vi "OE2012&OE2022_Configure Demodulator Filter.vi"(7 "OE2012&OE2022_\nConfigure Demod Filter":T1={"Time Constant(s) "=0.1, "Low Pass Filter Slope "=1, "Enable Sync Filter "=0, "Demodulator Source"=0, "Demodulator"=1} {"Demodulator" items=["Demod1"=1, "Demod2"=2, "Demod3"=3, "Demod4"=4, "Demod5"=5, "Demod6"=6, "Demod7"=7, "Demod8"=8]; "Demodulator Source" items=["Signal In 1", "Signal In 2", "Aux In 1", "Aux In 2", "Aux In 3", "Aux In 4", "X-Demod1", "Y-Demod1", "R-Demod1", "Theta-Demod1", "X-Demod5", "Y-Demod5", "R-Demod5", "Theta-Demod5"]; "Enable Sync Filter" items=["OFF", "ON"]; "Low Pass Filter Slope" items=["6 dB/oct", "12 dB/oct", "18 db/oct", "24 dB/oct", "30 dB/oct", "36 dB/oct", "42 dB/oct", "48 dB/oct"]; "Time Constant(s)" min=1e-06 max=3000.0}, 8 "Error in (no error)":errorcluster caption="error out（no error）", 9 "Remote Mode":u16(ring)=1 items=["RS232"=1, "Ethernet"=3], 10 "Connection ID in":refnum<k5>, 11 "VISA resource name":refnum<visa-resource-name>) -> (0 "Error out":errorcluster caption="error out", 1 "Output String":string, 2 "Connection ID out":refnum<k5>, 3 "VISA resource  out":refnum<visa-resource-name>)   [LabVIEW 2011]
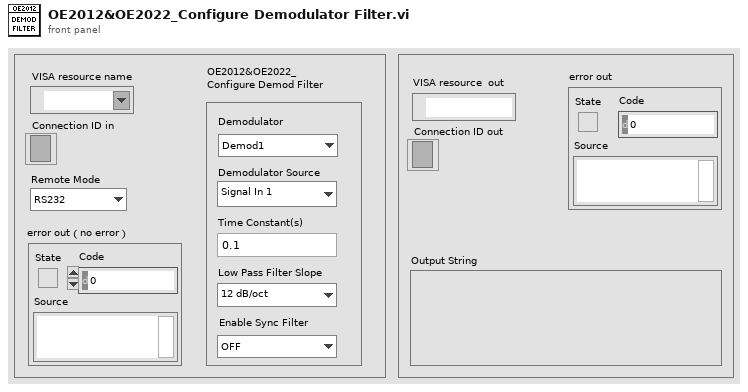
[diagram p1: front panel]
types:
  T1 = cluster{"Time Constant(s) ":dbl, "Low Pass Filter Slope ":u8, "Enable Sync Filter ":u16, "Demodulator Source":u16, "Demodulator":u16}
  T2 = enum16{"ISRC", "IGND", "ICPL", "ILIN", "PHAS", "FMOD", "RSLP", "FREQ", "SWPT", "SLLM", "SULM", "SSLL", "SSLG", "STLM", "SWRM", "IRNG", "SENS", "RMOD", "OFLT", "OFSL", "SYNC", "DMOD", "HARM", "DARB", "SWVT", "SLVL", "SVLL", "SVUL", "SVSL", "SVSG", "SVTM", "SVRM", "RALL", "SNAP", "OUTP", "OAUX", "COUT", "CAUX", "COFP", "CEXP", "FPOP", "OEXP", "*IDN", "*RST", "OVLD", "INOV", "GNOV", "*PLL", "SSET", "RSET", "AGAN", "APHS", "ARSV", "ASCL", "EQCD", "EQCS", "SPED", "SRAT", "SLEN", "SSLE", "STRG", "SPRM", "STRD", "PAUS", "REST", "SPTS", "TRCA", "TEMP", "RSTU", "IHNZ", "DEQU", "SADD", "ARNG", "CSPE", "ISRCD", "IGNDD", "ICPLD", "ILIND", "PHASD", "FMODD", "RSLPD", "FREQD", "SWPTD", "SLLMD", "SULMD", "SSLLD", "SSLGD", "STLMD", "SWRMD", "SENSD", "RMODD", "OFLTD", "OFSLD", "SYNCD", "HARMD", "EQCDD", "EQCSD", "SNAPD", "OUTPD", "SWVTD", "SLVLD", "SVLLD", "SVULD", "SVSLD", "SVSGD", "SVTMD", "SVRMD", "SVDCD", "ARSVD", "AGAND", "APHSD", "ASCLD", "FPOPD", "CAUXD", "OEXPD", "SPEDD", "SRATD", "SLEND", "SSLED", "STRGD", "SPRMD", "STRDD", "PAUSD", "RESTD", "SPTSD", "TRCAD", "*IDND", "*RSTD", "INOVD", "GNOVD", "*PLLD", "SSETD", "RSETD"}
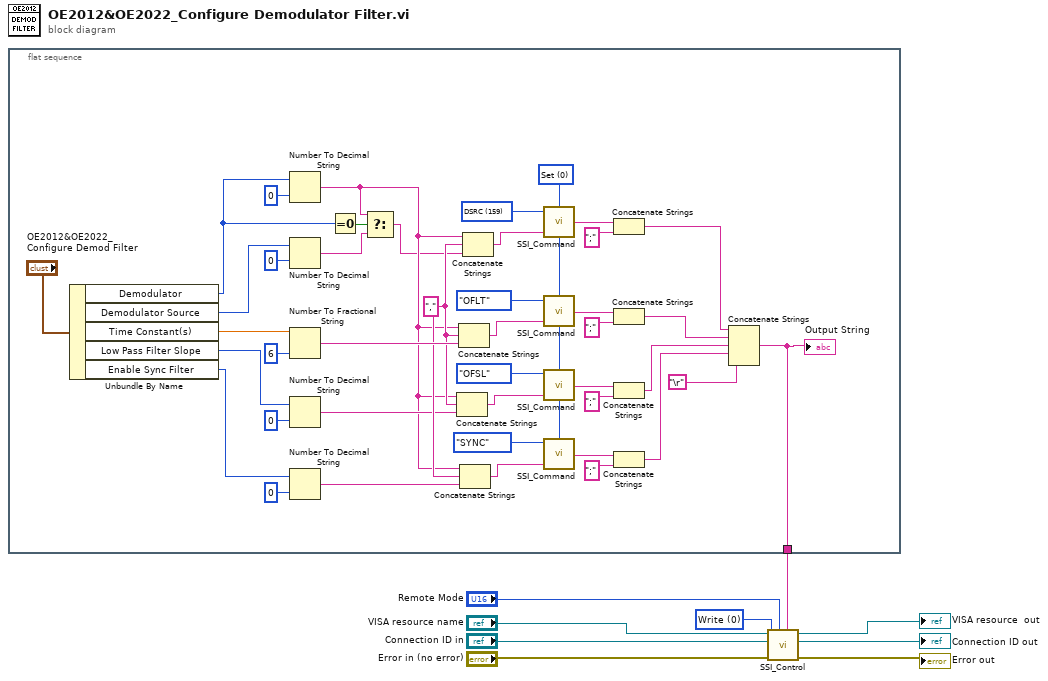
[diagram p0: block diagram]
diagram:
  w7 = u16 0 items=["Write", "Read"] ("Control")
  n1 = flat-sequence {
    tunnel: [w14] -> w1
    frame #0 {
      w18 = ","
      w26 = u16 159 items=["ISRC", "IGND", "ICPL", "ILIN", "PHAS", "FMOD", "RSLP", "FREQ", "SWPT", "SLLM", "SULM", "SSLL", "SSLG", "STLM", "SWRM", "IRNG", "SENS", "RMOD", "OFLT", "OFSL", "SYNC", "DMOD", "HARM", "DARB", "SWVT", "SLVL", "SVLL", "SVUL", "SVSL", "SVSG", "SVTM", "SVRM", "RALL", "SNAP", "OUTP", "OAUX", "COUT", "CAUX", "COFP", "CEXP", "FPOP", "OEXP", "*IDN", "*RST", "OVLD", "INOV", "GNOV", "*PLL", "SSET", "RSET", "AGAN", "APHS", "ARSV", "ASCL", "EQCD", "EQCS", "SPED", "SRAT", "SLEN", "SSLE", "STRG", "SPRM", "STRD", "PAUS", "REST", "SPTS", "TRCA", "TEMP", "RSTU", "INHZ", "DEQU", "SADD", "ARNG", "CSPE", "ISRCD", "IGNDD", "ICPLD", "ILIND", "PHASD", "FMODD", "RSLPD", "FREQD", "SWPTD", "SLLMD", "SULMD", "SSLLD", "SSLGD", "STLMD", "SWRMD", "SENSD", "RMODD", "OFLTD", "OFSLD", "SYNCD", "HARMD", "EQCDD", "EQCSD", "SNAPD", "OUTPD", "SWVTD", "SLVLD", "SVLLD", "SVULD", "SVSLD", "SVSGD", "SVTMD", "SVRMD", "SVDCD", "ARSVD", "AGAND", "APHSD", "ASCLD", "FPOPD", "CAUXD", "OEXPD", "SPEDD", "SRATD", "SLEND", "SSLED", "STRGD", "SPRMD", "STRDD", "PAUSD", "RESTD", "SPTSD", "TRCAD", "*IDND", "*RSTD", "INOVD", "GNOVD", "*PLLD", "SSETD", "RSETD", "RALLD", "NIPA", "NSMA", "NGWA", "NMAC", "NMOD", "TRIG", "TRCB", "INHZD", "ISAMD", "IRAGD", "RRAGD", "SOFFD", "DMODD", "COUTD", "COFPD", "CEXPD", "ARNGD", "OAUXD", "TRIM", "SUITD", "SNHZD", "AOFSD", "RSRC", "FEXT", "FINT", "DSRC"] ("Command Type")
      w34 = u16 0 items=["Set", "Query"] ("Opera")
      n2 = Unbundle By Name("OE2012&OE2022_\nConfigure Demod Filter") -> ("Demodulator"=w24:u16, "Demodulator Source"=w42:u16, "Time Constant(s)"=w41:dbl, "Low Pass Filter Slope"=w40:u8, "Enable Sync Filter"=w33:u16)
      n3 = Number To Decimal String(number=w24, width (-)=i16 0 ("宽度(-)")) -> (decimal integer string=w12:string)
      n4 = Number To Decimal String(number=w42, width (-)=i16 0 ("宽度(-)")) -> (decimal integer string=w11:string)
      n5 = Number To Fractional String(number=w41, precision (6)=i16 6 ("宽度(-)")) -> (F-format string=w19:string)  [unwired: 2 in]
      n6 = Number To Decimal String(number=w40, width (-)=i16 0 ("精度(6)")) -> (decimal integer string=w17:string)
      n7 = Number To Decimal String(number=w33, width (-)=i16 0 ("精度(6)")) -> (decimal integer string=w16:string)
      n8 = Equal To 0?(x=w24) -> (x = 0?=w13:bool)
      n9 = Select(t=w12, s=w13, f=w11) -> (s? t:f=w10:string)
      n10 = Concatenate Strings(w12, w18, w17) -> (w21:string)
      n11 = Concatenate Strings(w12, w18, w19) -> (w22:string)
      n12 = Concatenate Strings(w12, w18, w16) -> (w20:string)
      n13 = Concatenate Strings(w12, w18, w10) -> (w23:string)
      n14 = call "SSI_Command.vi"("Opera"=w34, "Paramter"=w23, "Command Type"=w26) -> ("Output string"=w48:string)  [unwired: 1 in]
      n15 = call "SSI_Command.vi"("Opera"=w34, "Paramter"=w22, "Command Type"=T2."OFLT") -> ("Output string"=w44:string)  [unwired: 1 in]
      n16 = call "SSI_Command.vi"("Opera"=w34, "Paramter"=w21, "Command Type"=T2."OFSL") -> ("Output string"=w46:string)  [unwired: 1 in]
      n17 = call "SSI_Command.vi"("Opera"=w34, "Paramter"=w20, "Command Type"=T2."SYNC") -> ("Output string"=w35:string)  [unwired: 1 in]
      n18 = Concatenate Strings(w48, ";" ("替换字符串(\"\")")) -> (w15:string)
      n19 = Concatenate Strings(w44, ";" ("替换字符串(\"\")")) -> (w39:string)
      n20 = Concatenate Strings(w46, ";" ("替换字符串(\"\")")) -> (w38:string)
      n21 = Concatenate Strings(w35, ";" ("替换字符串(\"\")")) -> (w28:string)
      n22 = Concatenate Strings(w15, w39, w38, w28, "\r") -> (w14:string)
      "Output String" <- w14
    }
  }
  n23 = call "SSI_Control.vi"("Write Buffer"=w1, "Remote Mode"="Remote Mode", "Error in (no error)"="Error in (no error)", "Control"=w7, "Connection ID in"="Connection ID in", "VISA resource name"="VISA resource name") -> ("Error out"=→"Error out":errorcluster, "Connection ID out"=→"Connection ID out":refnum<k5>, "VISA resource  out"=→"VISA resource  out":refnum<visa-resource-name>)  [unwired: 2 in, 1 out]
